vi "ProcessComicDirectory.vi"() -> ()   [LabVIEW 2022 SP3]
panel:
  in  "Escape":bool
  out "Deleted Files":string[](array[string])
  in  "Working Folder":path
  out "Current Comic":path
  out "Iteration":i32
  out "size(s)":i32
  in  "Folder Path":path
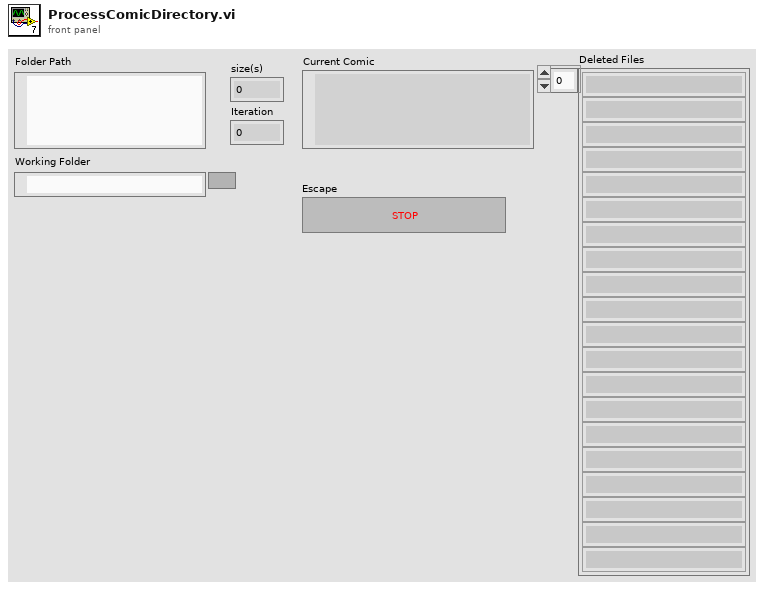
[diagram p1: front panel]
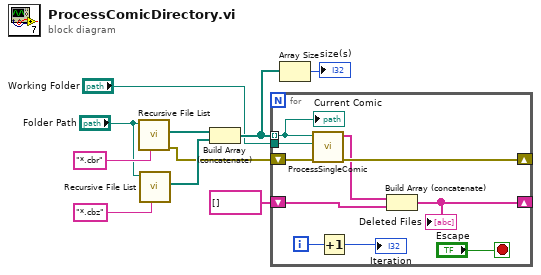
[diagram p0: block diagram]
diagram:
  n1 = call <vilib>:"Recursive File List.vi"("pattern"="*.cbr", "Folder Path"="Folder Path") -> ("error out"=w5:errorcluster, "All Files in Dir"=w7:path[])  [unwired: 5 in, 3 out]
  n2 = call <vilib>:"Recursive File List.vi"("pattern"="*.cbz", "Folder Path"="Folder Path") -> ("All Files in Dir"=w6:path[])  [unwired: 5 in, 4 out]
  n3 = Build Array (concatenate)(w7, w6) -> (w4:path[])
  n4 = for {
    tunnel: w4 -> [w19] mode=indexing
    shift-right: [w18] -> _
    shift-left: w5 -> [w20]
    tunnel: "Working Folder" -> [w16]
    shift-right: [w14] -> _
    shift-left: string[] [] -> [w15]
    i -> [w17]
    stop <- "Escape" stop-if-true
    n5 = call "ProcessSingleComic.vi"("error in"=w20, "Working Folder"=w16, "Original Comic File"=w19) -> ("error out"=w18:errorcluster, "Deleted files"=w13:string[])  [unwired: 7 in]
    n6 = Increment(x=w17) -> (x+1=→"Iteration":i32)
    n7 = Build Array (concatenate)(w13, w15) -> (w14:string[])
    "Deleted Files" <- w14
    "Current Comic" <- w19
  }
  n8 = Array Size(array=w4) -> (size(s)=→"size(s)":i32)
